vi "Grow.vi"(0 "object in":refnum<class "Snake.lvclass">, 1 "Coordinates":T1, 5 "error in (no error)":errorcluster) -> (14 "object out":refnum<class "Snake.lvclass">, 19 "error out":errorcluster)   [LabVIEW 2021, in "Snake.lvclass"]
uses:
  Snake.lvclass
  Coordinates.ctl
  Snake.lvclass/Snake.ctl
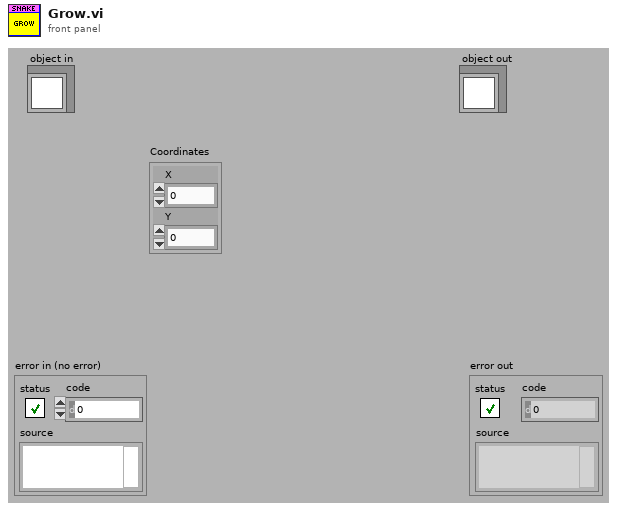
[diagram p1: front panel]
types:
  T1 = typedef "Coordinates.ctl" = cluster{"X":i32, "Y":i32}
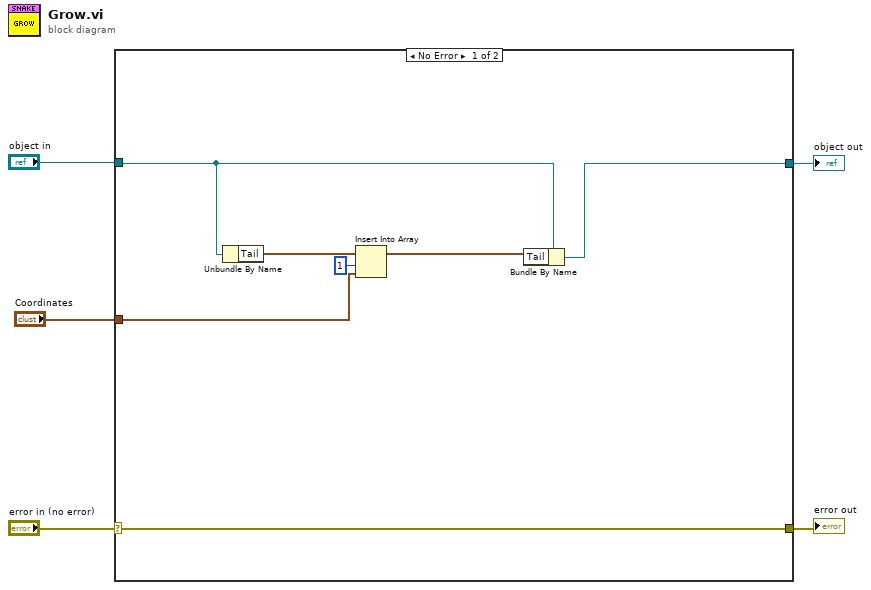
[diagram p0: block diagram]
diagram:
  n1 = case shown="No Error" "error in (no error)" {
    selector: "error in (no error)" -> [w12 w14]
    tunnel: [w12 w14] -> w4
    tunnel: [w10 w13] -> w2
    tunnel: "object in" -> [w11 w13]
    tunnel: "Coordinates" -> [w8 _]
    frame No Error {
      n2 = Unbundle By Name(w11) -> ("Tail"=w9:T1[])
      n3 = Insert Into Array(array=w9, index=1, new element=w8) -> (w6:T1[])
      n4 = Bundle By Name(cluster=w11, "Tail"=w6) -> (w10:refnum<class "Snake.lvclass">)
    }
    frame Error {
    }
  }
  "error out" <- w4
  "object out" <- w2
